vi "打印.vi"(8 "error in (no error)":errorcluster caption="错误输入（无错误）", 11 "eagle 输入":refnum<class "eagle.lvclass">) -> (0 "error out":errorcluster caption="错误输出", 2 "字符串":string, 3 "eagle 输出":refnum<class "eagle.lvclass">)   [LabVIEW 2020, in "eagle.lvclass"]
uses:
  eagle.lvclass
  Animal/Animal.lvclass
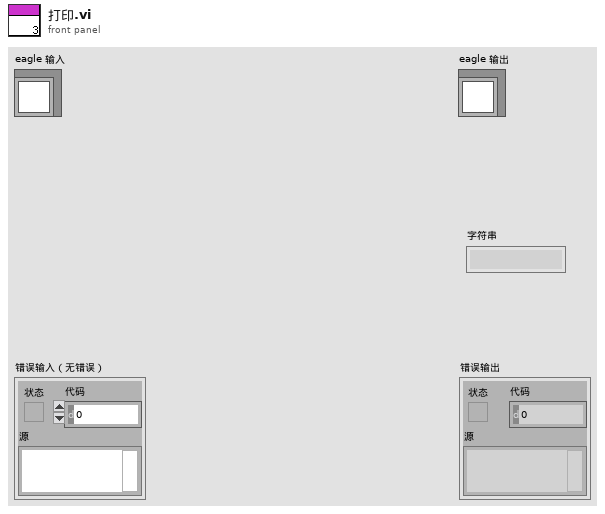
[diagram p1: front panel]
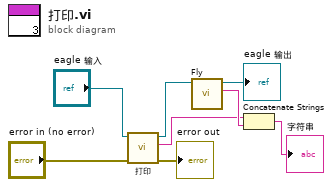
[diagram p0: block diagram]
diagram:
  n1 = call-parent "打印.vi"("error in (no error)"="error in (no error)", "Animal 输入"="eagle 输入") -> ("error out"=→"error out":errorcluster, "字符串"=w2:string, "Animal 输出"=w5:refnum<class "eagle.lvclass">)  [unwired: 7 in]
  n2 = call-dynamic "Fly.vi"("eagle 输入"=w5) -> ("字符串 2"=w3:string, "eagle 输出"=→"eagle 输出":refnum<class "eagle.lvclass">)  [unwired: 8 in, 1 out]
  n3 = Concatenate Strings(w2, w3) -> (→"字符串":string)
